vi "Write set period.vi"(8 "error in":errorcluster, 10 "set period":bool, 11 "timing source in":refnum<class "scan engine timing source.lvclass">) -> (0 "error out":errorcluster, 3 "timing source out":refnum<class "scan engine timing source.lvclass">)   [LabVIEW 2013, in "scan engine timing source.lvclass"]
doc: "Overwrites the <b>set period</b> flag in the object. If it is, initialize will set the period of the scan engine. If false, the period will not be set. By default, the write scan period method will set this flag."
uses:
  scan engine timing source.lvclass
  scan engine timing source.lvclass/scan engine timing source.ctl
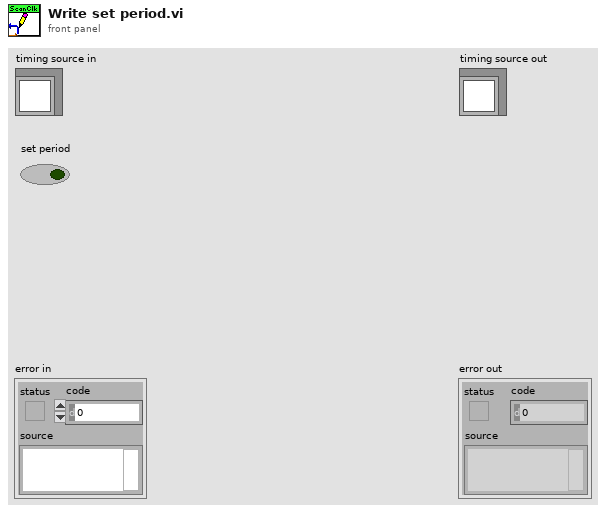
[diagram p1: front panel]
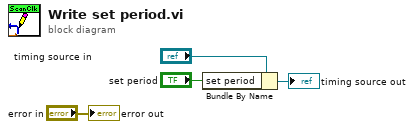
[diagram p0: block diagram]
diagram:
  n1 = Bundle By Name(cluster="timing source in", "set period"="set period") -> (→"timing source out":refnum<class "scan engine timing source.lvclass">)
  "error out" <- "error in"
